vi "Force Channel.vi"(6 "timeout (ms)":i32=5000, 8 "error in":errorcluster, 10 "Force Channel":T1, 11 "gRPC ID":T2) -> (0 "error out":errorcluster, 3 "gRPC ID out":T2)   [LabVIEW 2021, in "CIFCoreWrapper.lvlib"]
uses:
  CIFCoreWrapper.lvlib
  CIFCoreChannel_client/CIFCoreChannel_client.lvlib
  <vilib>/gRPC/LabVIEW gRPC Library/Shared/grpcId.ctl
  <vilib>/gRPC/LabVIEW gRPC Library/grpc-lvsupport-release.lvlib
  CIFCoreChannel_client/RPC Messages/cif_channelcore_SetForceRequest.ctl
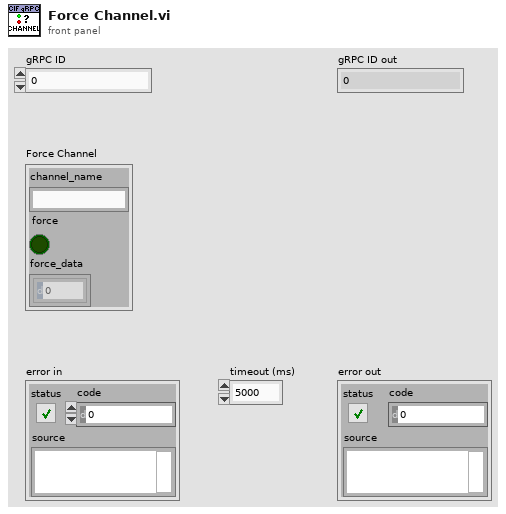
[diagram p1: front panel]
types:
  T1 = typedef "CIFCoreChannel_client.lvlib/cif_channelcore_SetForceRequest.ctl" = cluster{"channel_name":string, "force":bool, "force_data":u8[]}
  T2 = typedef "grpc-lvsupport-release.lvlib/grpcId.ctl" = u64
  T3 = typedef "CIFCoreChannel_client.lvlib/cif_channelcore_SetForceResponse.ctl" = cluster{"status":T4}
  T4 = typedef "CIFCoreChannel_client.lvlib/cif_common_Status.ctl" = cluster{"code":i32, "message":string}
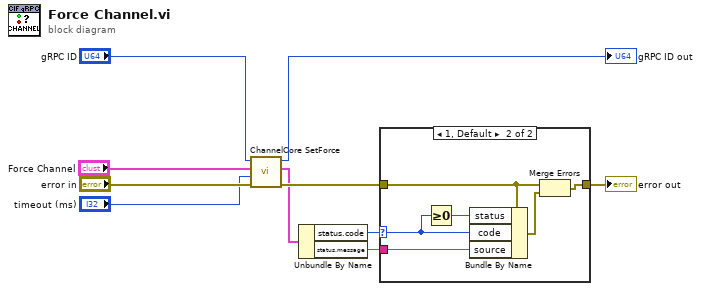
[diagram p0: block diagram]
diagram:
  n1 = call "ChannelCore SetForce.vi"("error in"="error in", "timeout (ms)"="timeout (ms)", "Request Data"="Force Channel", "gRPC ID"="gRPC ID") -> ("error out"=w5:errorcluster, "Response Data"=w2:T3, "gRPC ID out"=→"gRPC ID out":T2)  [unwired: 5 in]
  n2 = Unbundle By Name(w2) -> ("status.code"=w3:i32, "status.message"=w6:string)
  n3 = case shown="1, Default" w3 {
    selector: w3 -> [_ w12]
    tunnel: w6 -> [_ w16]
    tunnel: w5 -> [w11 w15]
    tunnel: [w11 w13] -> w4
    frame 0 {
    }
    frame 1, Default {
      n4 = Greater Or Equal To 0?(x=w12) -> (x >= 0?=w17:bool)
      n5 = Bundle By Name(cluster=w15, "status"=w17, "code"=w12, "source"=w16) -> (w14:errorcluster)
      n6 = Merge Errors(w15, w14) -> (w13:errorcluster)
    }
  }
  "error out" <- w4
